vi "outputSettings.vi"(8 "所有串口":string[](array[string]), 9 "执行:调用时显示前面板":bool, 11 "电压脉冲卡选择":string[](array[string])) -> (0 "串口电流服务选定口":string[](array[string]), 1 "电流源串口选定":string[](array[string]), 2 "电压脉冲开关 2":bool, 3 "电压脉冲卡选":u16, 4 "波特率set":u32)   [LabVIEW 2020]
panel:
  in  "电流源表2：":u16(ring) items=["No Select COM", "ASRL1::INSTR", "ASRL2::INSTR", "ASRL10::INSTR"]
  in  "电流源表1：":u16(ring) items=["No Select COM", "ASRL1::INSTR", "ASRL2::INSTR", "ASRL10::INSTR"]
  in  "串口电流值服务2：":u16(ring) items=["No Select COM", "ASRL1::INSTR", "ASRL2::INSTR", "ASRL10::INSTR"]
  out "面板开":bool
  in  "波特率：":u32=57600
  in  "串口电流值服务1：":u16(ring) items=["No Select COM", "ASRL1::INSTR", "ASRL2::INSTR", "ASRL10::INSTR"]
  in  "电压脉冲开关：":bool
  in  "电压脉冲卡选择：":u16(ring) items=["NI Simulated DAQ Device-0"]
  # "电压输出"
  # "电流源表"
  # "有电流源表时,仅设置此栏串口号,且不可相同。电流表波特率必须为57600。"
  # "串口电流"
  # "无电流源表时,方可设置此栏串口号,且不可相同。"
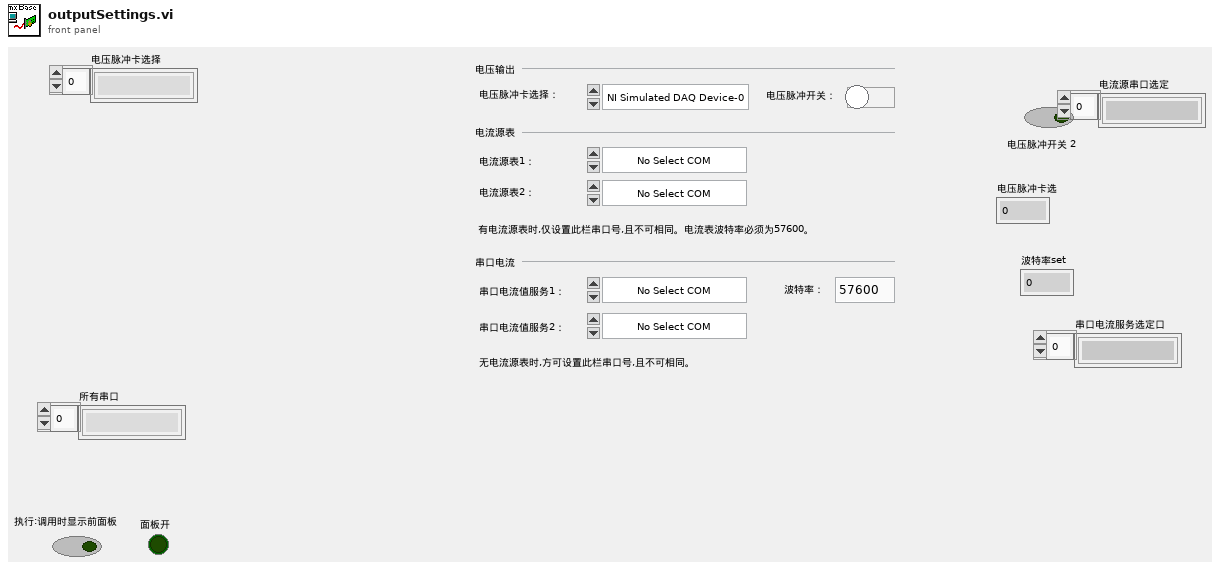
[diagram p1: front panel]
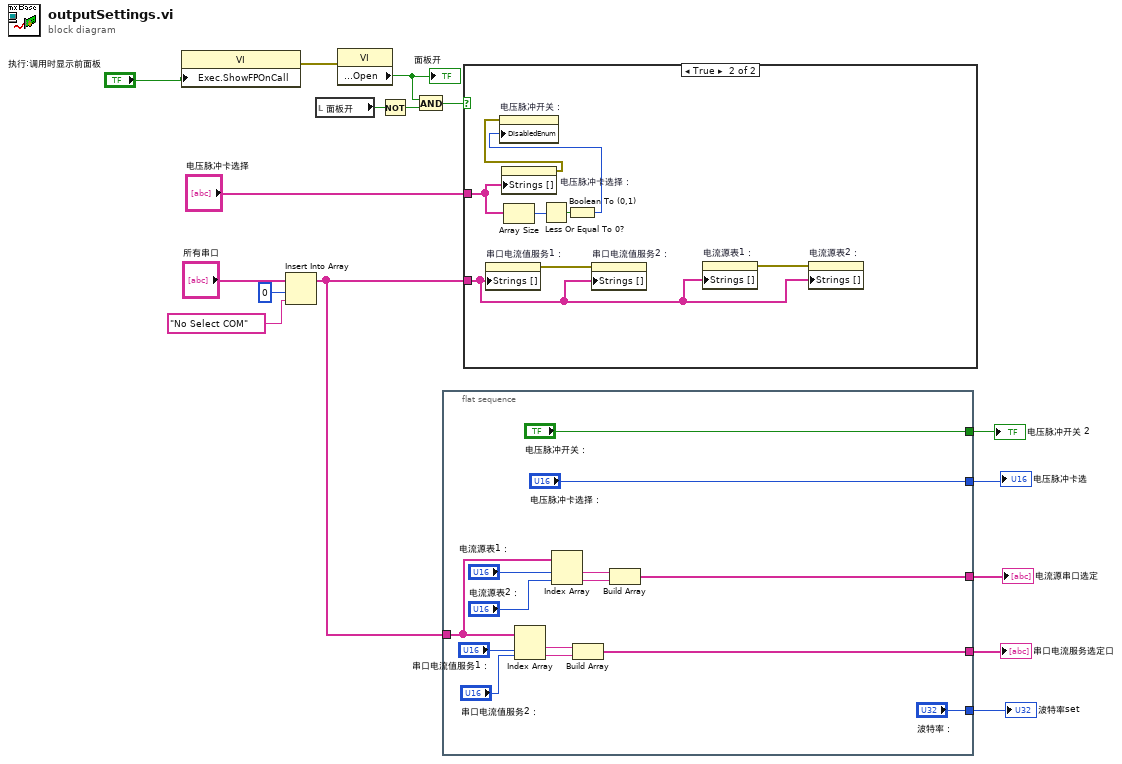
[diagram p0: block diagram]
diagram:
  n1 = property class="VI"("Exec.ShowFPOnCall"="执行:调用时显示前面板") -> (error out=w14:errorcluster)  [unwired: 2 in, 1 out]
  n2 = Insert Into Array(array="所有串口", index=0 ("索引"), new element="No Select COM" ("新元素/子数组")) -> (w4:string[])
  n3 = local read "面板开"() -> (w13:bool)
  n4 = property class="VI"(error in=w14) -> ("Front Panel.Open"=w11:bool)  [unwired: 1 in, 2 out]
  "面板开" <- w11
  n5 = Not(x=w13) -> (.not. x?=w12:bool)
  n6 = And(x=w11, y=w12) -> (x .and. y?=w10:bool)
  n7 = flat-sequence {
    tunnel: ["电压脉冲开关："] -> w16
    tunnel: [w17] -> w1
    tunnel: ["波特率："] -> w5
    tunnel: w4 -> [w20]
    tunnel: [w24] -> w9
    tunnel: ["电压脉冲卡选择："] -> w2
    frame #0 {
      n8 = Index Array(array=w20, index #1="串口电流值服务1：", index #2="串口电流值服务2：") -> (element #1=w26:string, element #2=w25:string)
      n9 = Index Array(array=w20, index #1="电流源表1：", index #2="电流源表2：") -> (element #1=w19:string, element #2=w18:string)
      n10 = Build Array(w26, w25) -> (w24:string[])
      n11 = Build Array(w19, w18) -> (w17:string[])
    }
  }
  n12 = case shown="True" w10 {
    tunnel: "电压脉冲卡选择" -> [_ w36]
    tunnel: w4 -> [_ w31]
    frame False {
    }
    frame True {
      n13 = property on="串口电流值服务1：" class="Ring (strict)"("Strings []"=w31) -> (error out=w35:errorcluster)  [unwired: 2 in, 1 out]
      n14 = property on="电压脉冲卡选择：" class="Ring (strict)"("Strings []"=w36) -> (error out=w34:errorcluster)  [unwired: 2 in, 1 out]
      n15 = Array Size(array=w36) -> (size(s)=w38:i32)
      n16 = Less Or Equal To 0?(x=w38) -> (x <= 0?=w37:bool)
      n17 = Boolean To (0,1)(Boolean=w37) -> (0, 1=w33:i16)
      n18 = property on="电压脉冲开关：" class="Bool (strict)"(error in=w34, "DisabledEnum"=w33) -> ()  [unwired: 1 in, 2 out]
      n19 = property on="串口电流值服务2：" class="Ring (strict)"(error in=w35, "Strings []"=w31) -> ()  [unwired: 1 in, 2 out]
      n20 = property on="电流源表1：" class="Ring (strict)"("Strings []"=w31) -> (error out=w32:errorcluster)  [unwired: 2 in, 1 out]
      n21 = property on="电流源表2：" class="Ring (strict)"(error in=w32, "Strings []"=w31) -> ()  [unwired: 1 in, 2 out]
    }
  }
  "电压脉冲开关 2" <- w16
  "串口电流服务选定口" <- w9
  "波特率set" <- w5
  "电压脉冲卡选" <- w2
  "电流源串口选定" <- w1
